vi "Load Snapshot.vi"(6 "IPath Getter in":refnum<class "IPath Getter.lvclass">, 8 "error in":errorcluster, 10 "Debug Elements Options":T1={"Breakpoints"=TRUE, "Probes"=TRUE}, 11 "VI Reference in":refnum<vi>) -> (0 "error out":errorcluster, 2 "VI Modified":bool, 3 "VI Reference out":refnum<vi>)   [LabVIEW 2020, in "Public API.lvlib"]
doc: "Load <b>Debug Snapshot</b> (i.e. breakpoints and probes) and apply them to the active VI."
uses:
  Public API.lvlib
  Type Definitions/Snapshot Handling Options--cluster.ctl
  IPath Getter/IPath Getter.lvclass
  Type Definitions/Class Name--enum.ctl
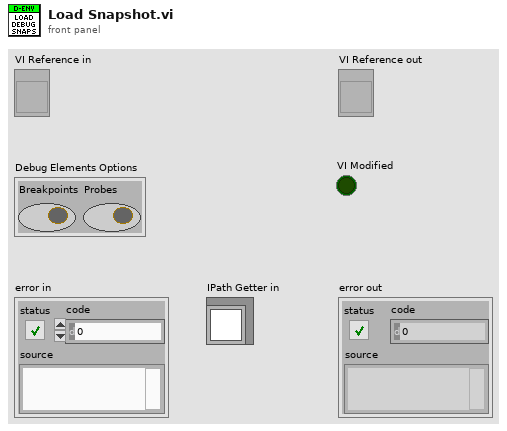
[diagram p1: front panel]
types:
  T1 = typedef "Snapshot Handling Options--cluster.ctl" = cluster{"Breakpoints":bool, "Probes":bool}
  T2 = typedef "Class Name--enum.ctl" = enum16{"Node", "Wire"}
  T3 = typedef "Debug Snapshot--cluster.ctl" = cluster{"VI Name":string, "Breakpoints":T4[], "Probes":i32[]}
  T4 = typedef "Breakpoint--cluster.ctl" = cluster{"UID":i32, "BP Status":T5, "Class Name":T2}
  T5 = typedef "LVBreakpointStatusEnum.ctl" = enum8{"Cleared Break", "Enabled Break", "Disabled Break"}
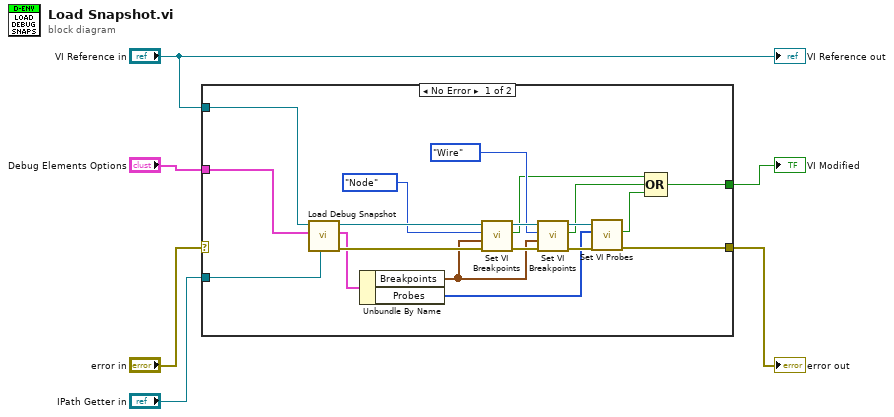
[diagram p0: block diagram]
diagram:
  n1 = case shown="No Error" "error in" {
    selector: "error in" -> [_ w26]
    tunnel: "VI Reference in" -> [w21 _]
    tunnel: "Debug Elements Options" -> [w20 _]
    tunnel: [w22 w26] -> w5
    tunnel: [w8 _] -> w2
    tunnel: "IPath Getter in" -> [w7 _]
    frame No Error {
      n2 = call "Load Debug Snapshot.vi"("IPath Getter in"=w7, "Debug Elements Options"=w20, "VI Reference in"=w21) -> ("error out"=w25:errorcluster, "VI Debug Elements"=w15:T3, "VI Reference out"=w19:refnum<vi>)  [unwired: 6 in]
      n3 = Unbundle By Name(w15) -> ("Breakpoints"=w14:T4[], "Probes"=w13:i32[])
      n4 = call "Set VI Breakpoints.vi"("error in"=w25, "Breakpoints"=w14, "Class Name"=Class_Name--enum."Node", "VI Reference in"=w19) -> ("error out"=w24:errorcluster, "VI Modified"=w9:bool, "VI Reference out"=w18:refnum<vi>)  [unwired: 5 in]
      n5 = call "Set VI Breakpoints.vi"("error in"=w24, "Breakpoints"=w14, "Class Name"=Class_Name--enum."Wire", "VI Reference in"=w18) -> ("error out"=w23:errorcluster, "VI Modified"=w10:bool, "VI Reference out"=w12:refnum<vi>)  [unwired: 5 in]
      n6 = call "Set VI Probes.vi"("error in"=w23, "Probes"=w13, "VI Reference in"=w12) -> ("error out"=w22:errorcluster, "VI Modified"=w11:bool)  [unwired: 6 in, 1 out]
      n7 = Compound Arithmetic op=OR(w9, w10, w11) -> (w8:bool)
    }
    frame Error {
      # "Pass error without further action"
    }
  }
  "error out" <- w5
  "VI Modified" <- w2
  "VI Reference out" <- "VI Reference in"
